vi "set-temperature.vi"(9 "输出数值":cluster{"温度阈值":dbl, "亮度阈值":dbl, "电源阈值":dbl}, 10 "数值":sgl, 11 "字符串输入":string) -> (3 "字符串输出":string)   [LabVIEW 2012]
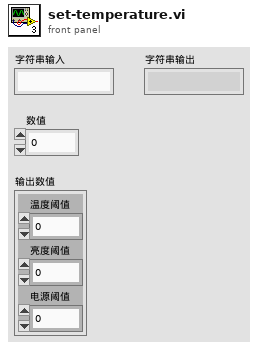
[diagram p1: front panel]
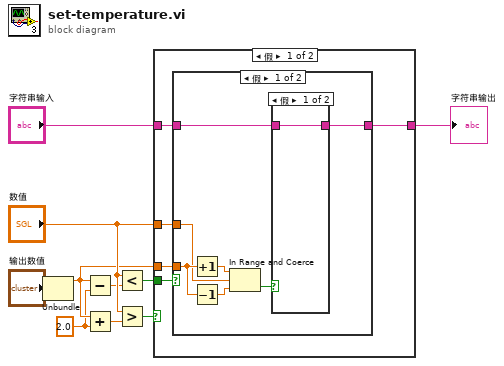
[diagram p0: block diagram]
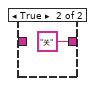
[diagram p2: hidden frame]
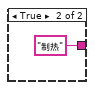
[diagram p3: hidden frame]
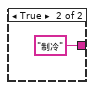
[diagram p4: hidden frame]
diagram:
  w3 = 2.0 ("y")
  n1 = Unbundle("输出数值") -> ("温度阈值"=w8:dbl)  [unwired: 2 out]
  n2 = Subtract(x=w8, y=w3) -> (x-y=w6:dbl)
  n3 = Add(x=w8, y=w3) -> (x+y=w2:dbl)
  n4 = Less?(x="数值", y=w6) -> (x < y?=w7:bool)
  n5 = Greater?(x="数值", y=w2) -> (0:w4:bool)
  n6 = case shown="假" w4 {
    tunnel: [w14 "制冷"] -> w5
    tunnel: w7 -> [w15 _]
    tunnel: w8 -> [w13 _]
    tunnel: "数值" -> [w12 _]
    tunnel: "字符串输入" -> [w11 _]
    frame False {
      n7 = case shown="假" w15 {
        tunnel: [w17 "制热"] -> w14
        tunnel: w13 -> [w20 _]
        tunnel: w12 -> [w19 _]
        tunnel: w11 -> [w16 _]
        frame False {
          n8 = Increment(x=w20) -> (x+1=w21:dbl)
          n9 = Decrement(x=w20) -> (x-1=w22:dbl)
          n10 = In Range and Coerce(upper limit=w21, x=w19, lower limit=w22) -> (In Range?=w18:bool)  [unwired: 1 out]
          n11 = case shown="假" w18 {
            tunnel: [w23 "关"] -> w17
            tunnel: w16 -> [w23 _]
            frame False {
            }
            frame True {
            }
          }
        }
        frame True {
        }
      }
    }
    frame True {
    }
  }
  "字符串输出" <- w5
